vi "_PC_MS_SubVI updateSysValue.vi"(8 "error in (no error)":errorcluster, 10 "sys_value_param":T1, 11 "sys_value_list":refnum<vi>) -> (0 "error out":errorcluster)   [LabVIEW 2018]
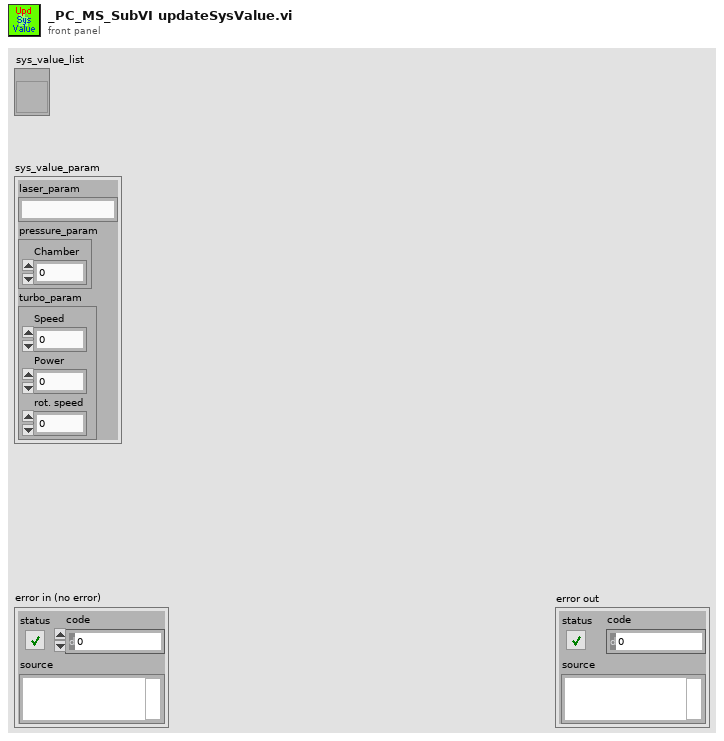
[diagram p1: front panel]
types:
  T1 = cluster{"laser_param":string, "pressure_param":cluster{"Chamber":dbl}, "turbo_param":cluster{"Speed":dbl, "Power":dbl, "rot. speed":dbl}}
  T2 = cluster{"Speed":dbl, "Power":dbl, "rot. speed":dbl}
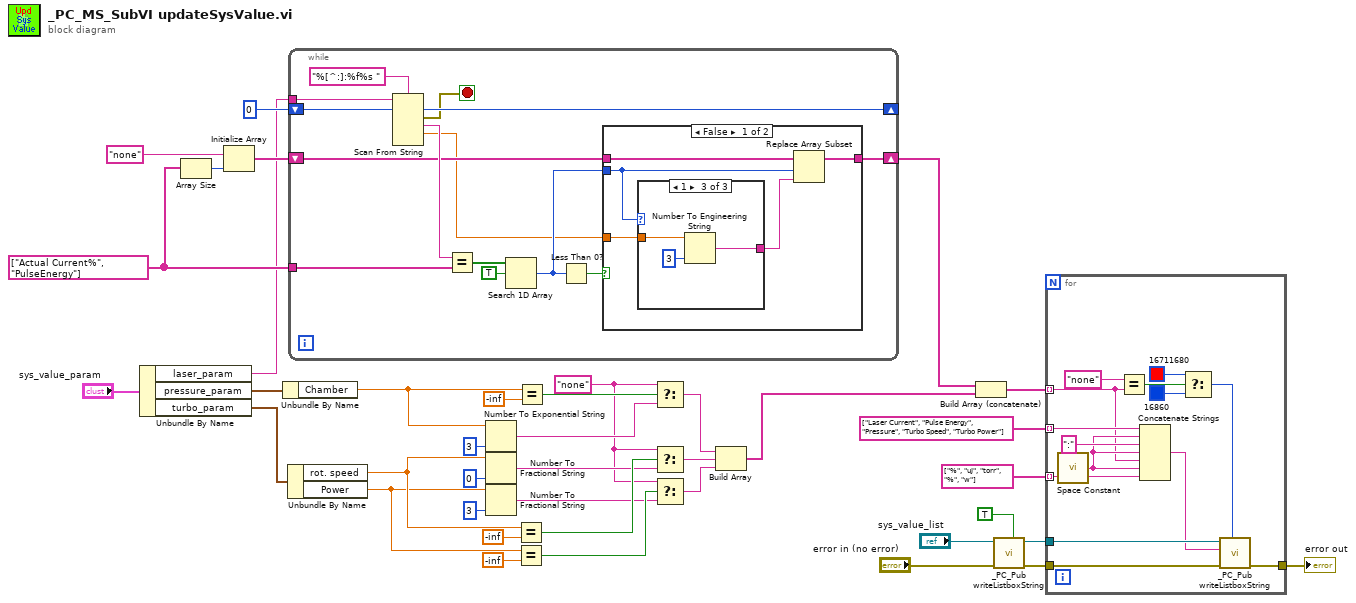
[diagram p0: block diagram]
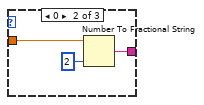
[diagram p3: hidden frame]
diagram:
  w11 = "none" ("t")
  w37 = string[] ["Actual Current%", "PulseEnergy"]
  n1 = Unbundle By Name("sys_value_param") -> ("laser_param"=w19:string, "pressure_param"=w6:cluster{"Chamber":dbl}, "turbo_param"=w32:T2)
  n2 = Array Size(array=w37) -> (size(s)=w36:i32)
  n3 = Initialize Array("none", w36) -> (w35:string[])
  n4 = Unbundle By Name(w6) -> ("Chamber"=w5:dbl)
  n5 = Unbundle By Name(w32) -> ("rot. speed"=w17:dbl, "Power"=w16:dbl)
  n6 = while {
    shift-right: [w52] -> _
    shift-left: u32 0 -> [w51]
    tunnel: w19 -> [w49]
    tunnel: w37 -> [w47]
    shift-right: [w42] -> w31
    shift-left: w35 -> [w43]
    stop <- w50 stop-if-true
    n7 = Scan From String(format string="%[^:]:%f%s ", input string=w49, initial scan location=w51) -> (offset past scan=w52:u32, error out=w50:errorcluster, output 1=w48:string, output 2=w40:dbl)  [unwired: 5 in, 1 out]
    n8 = Equal?(x=w48, y=w47) -> (x = y?=w46:bool[])
    n9 = Search 1D Array(1D array=w46, element=TRUE) -> (index of element=w41:i32)  [unwired: 1 in]
    n10 = Less Than 0?(x=w41) -> (x < 0?=w44:bool)
    n11 = case shown="False" w44 {
      tunnel: w43 -> [w58 w65]
      tunnel: [w57 w65] -> w42
      tunnel: w41 -> [w56 _]
      tunnel: w40 -> [w55 _]
      frame False {
        n12 = case shown="1" w56 {
          tunnel: w55 -> [_ w61 w64]
          tunnel: [_ w59 w63] -> w54
          frame -1, Default {
          }
          frame 0 {
            n13 = Number To Fractional String(number=w61, precision (6)=i16 2) -> (F-format string=w59:string)  [unwired: 2 in]
          }
          frame 1 {
            n14 = Number To Engineering String(2:i16 3 ("precision (6)"), 4:w64) -> (0:w63:string)  [unwired: 2 in]
          }
        }
        n15 = Replace Array Subset(array=w58, new element=w54, index=w56) -> (w57:string[])
      }
      frame True {
      }
    }
  }
  n16 = Number To Exponential String(number=w5, precision (6)=i16 3) -> (E-format string=w18:string)  [unwired: 2 in]
  n17 = Number To Fractional String(number=w17, precision (6)=i16 0) -> (F-format string=w13:string)  [unwired: 2 in]
  n18 = Number To Fractional String(number=w16, precision (6)=i16 3) -> (F-format string=w12:string)  [unwired: 2 in]
  n19 = Equal?(x=w17, y=-inf) -> (x = y?=w15:bool)
  n20 = Equal?(x=w16, y=-inf) -> (x = y?=w14:bool)
  n21 = Equal?(x=w5, y=-inf) -> (x = y?=w20:bool)
  n22 = Select(t=w11, s=w20, f=w18) -> (s? t:f=w10:string)
  n23 = Select(t=w11, s=w15, f=w13) -> (s? t:f=w9:string)
  n24 = Select(t=w11, s=w14, f=w12) -> (s? t:f=w8:string)
  n25 = Build Array(w10, w9, w8) -> (w7:string[])
  n26 = Build Array (concatenate)(w31, w7) -> (w30:string[])
  n27 = call "_PC_Pub writeListboxString.vi"("Reset (F)"=TRUE, "error in (no error)"="error in (no error)", "Listbox Ref Input"="sys_value_list") -> ("error out"=w26:errorcluster, "Listbox Ref Output"=w27:refnum<vi>)  [unwired: 7 in]
  n28 = for {
    tunnel: w30 -> [w72] mode=indexing
    tunnel: string[] ["Laser Current", "Pulse Energy", "Pressure", "Turbo Speed", "Turbo Power"] -> [w75] mode=indexing
    tunnel: string[] ["%", "uJ", "torr", "%", "w"] -> [w66] mode=indexing
    tunnel: w27 -> [w79]
    tunnel: w26 -> [w78]
    tunnel: [w76] -> w25
    n29 = call <vilib>:"Space Constant.vi"() -> ("String"=w73:string)
    n30 = Equal?(x="none", y=w72) -> (x = y?=w70:bool)
    n31 = Concatenate Strings(w75, w73, ":" ("string"), w73, w72, w73, w66) -> (w77:string)
    n32 = Select(t=u32 16711680 ("String Color"), s=w70, f=u32 16860 ("String Color")) -> (s? t:f=w67:u32)
    n33 = call "_PC_Pub writeListboxString.vi"("String Color"=w67, "error in (no error)"=w78, "update_Str"=w77, "Listbox Ref Input"=w79) -> ("error out"=w76:errorcluster)  [unwired: 6 in, 1 out]
  }
  "error out" <- w25
